vi "Read Value at Path(String).vi"(8 "error in (no error)":errorcluster, 10 "Path String":string, 11 "Variant in":variant) -> (0 "error out":errorcluster, 2 "Element out":variant, 3 "Variant out":variant)   [LabVIEW 2017, in "Variant Data Manipulation.lvlib"]
uses:
  Variant Data Manipulation.lvlib
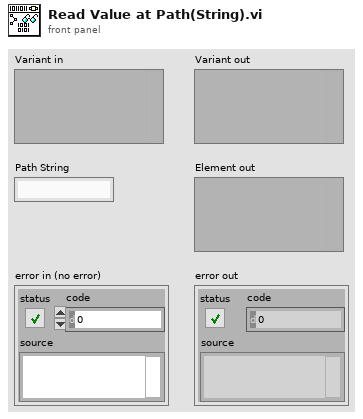
[diagram p1: front panel]
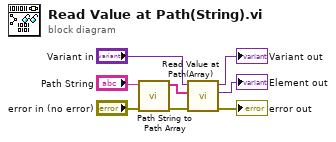
[diagram p0: block diagram]
diagram:
  n1 = call "Path String to Path Array.vi"("error in (no error)"="error in (no error)", "Path String"="Path String") -> ("error out"=w7:errorcluster, "Path Array"=w8:string[])  [unwired: 8 in]
  n2 = call "Read Value at Path(Array).vi"("error in (no error)"=w7, "Path in"=w8, "Variant in"="Variant in") -> ("error out"=→"error out":errorcluster, "Element out"=→"Element out":variant, "Variant out"=→"Variant out":variant)  [unwired: 6 in]
